vi "Enqueue.vi"   [LabVIEW 2019, in "Message Queue.lvlib"]
uses:
  Message Queue.lvlib
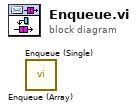
[diagram p0: block diagram]
diagram:
  n1 = call "Enqueue (Array).vi"() -> ()  [unwired: 10 in, 2 out]
  n2 = call "Enqueue (Single).vi"() -> ()  [unwired: 10 in, 2 out]
